vi "XMenuBar-Facade.vi"(0 "Data In":T5, 2 "Display State In":T3, 3 "Container State":T4) -> (6 "Data Out":T5, 7 "Display State Out":T3, 8 "Action":T2)   [LabVIEW 2020, in "XMenuBar.xctl"]
uses:
  XMenuBar.xctl
  XMenuBar-Data.ctl
  CMenu/CMenu.lvclass
  <vilib>/_xctls/Container State.ctl
  XMenuBar-State.ctl
  <vilib>/_xctls/Action.ctl
  Ctrls/black-Sel.ctl
  XSubMenu/XSubMenu.xctl
  <vilib>/_xctls/XControlSupport.lvlib
panel:
  in  "XSubMenu2":i32(xcontrol)
  in  "XSubMenu":i32(xcontrol)
  in  "Sel":T1
  out "MenuBar":string[](array[string])
  in  "BarBg":bool
  # "1. Drop the controls that make up the appearance\nof the XControl here.\n\n2. Resize the window to fit the controls\n\n3. If the XControl is of fixed size,  make the \n window not resizable from VI Properties->Window Appearance.\n\n4. If you want the controls to automatically size when the XControl sizes, check  \"Scale all objects on front panel when window resizes\" in File->VI Properties->Window Size page.\n\n5. Show the block diagram and handle events for the controls on this panel."
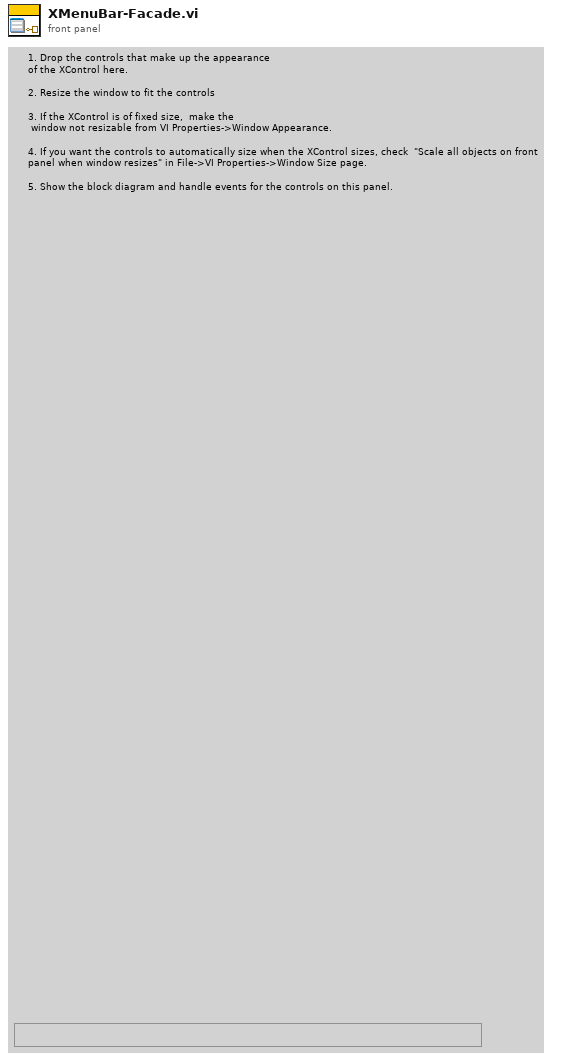
[diagram p1: front panel]
types:
  T1 = typedef "black-Sel.ctl" = bool
  T2 = typedef "XControlSupport.lvlib/Action.ctl" = cluster{"Data Changed?":bool, "State Changed?":bool, "Action Name":string}
  T3 = typedef "XMenuBar.xctl/XMenuBar-State.ctl" = cluster{"MenuFilePath":path}
  T4 = typedef "XControlSupport.lvlib/Container State.ctl" = cluster{"Indicator?":bool, "Run Mode?":bool, " Refnum":refnum<vi>}
  T5 = typedef "XMenuBar.xctl/XMenuBar-Data.ctl" = refnum<class "CMenu.lvclass">
  T6 = cluster{"Tag":string, "Name":string, "Symbol":i32, "Checked":bool, "ParentTag":string}[]
  T7 = enum16{"open", "replace", "create", "open or create", "replace or create", "replace or create with confirmation"}
  T8 = cluster{"Tag":string, "Name":string, "Symbol":i32, "Checked":bool, "ParentTag":string}
  T9 = cluster{"Tag":string, "Caption":string, "Symbol":i32, "Checked":bool, "OwnerTag":string}[]
  T10 = cluster{"Tag":string, "Name":string, "Index":i32, "Checked":bool, "Parent":string}[]
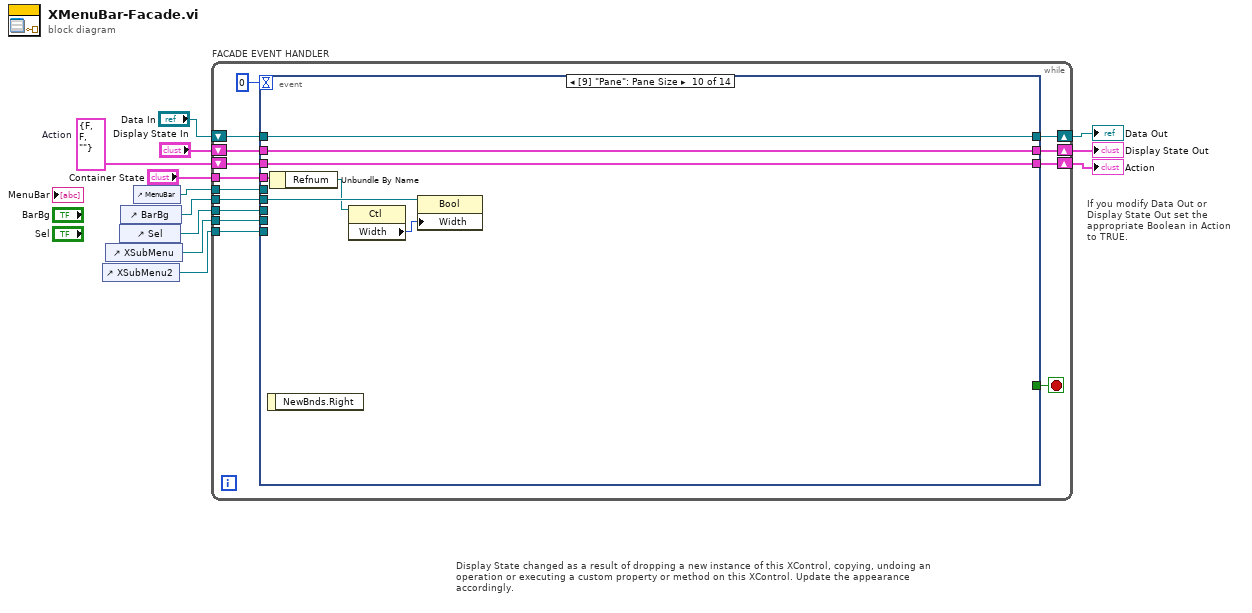
[diagram p0: block diagram]
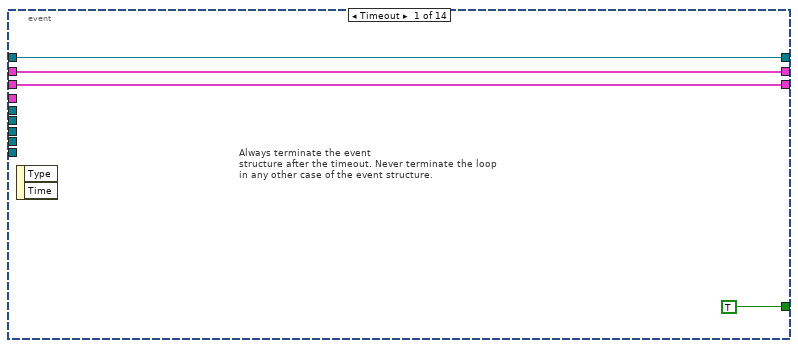
[diagram p2: hidden frame]
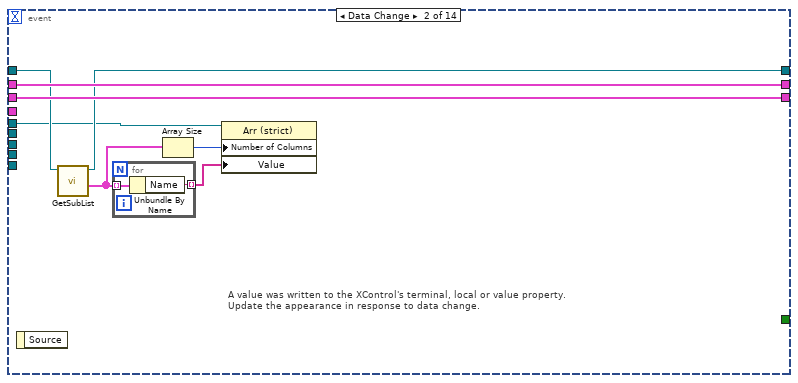
[diagram p3: hidden frame]
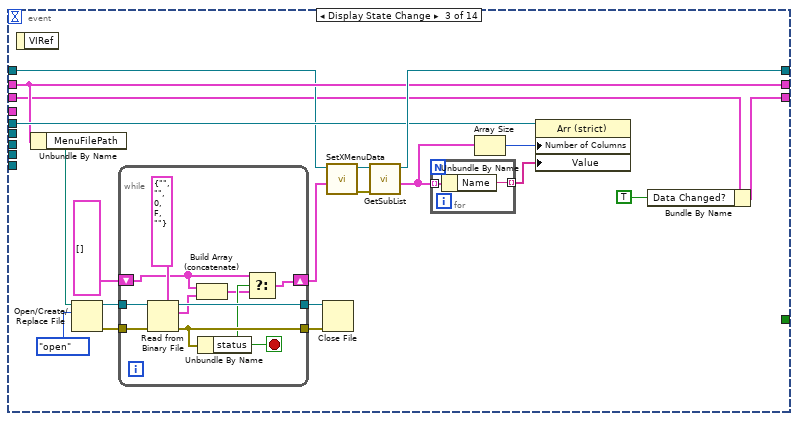
[diagram p4: hidden frame]
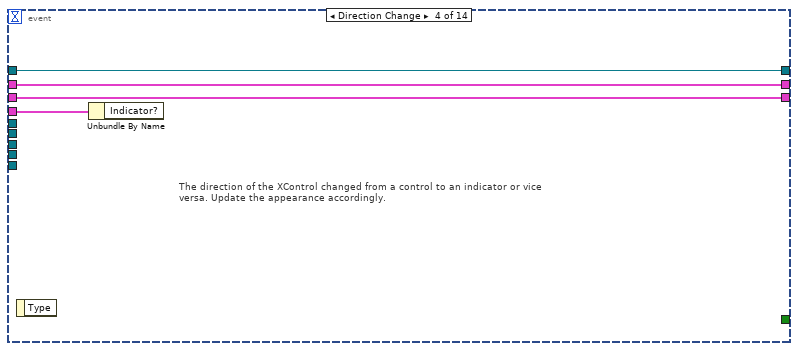
[diagram p5: hidden frame]
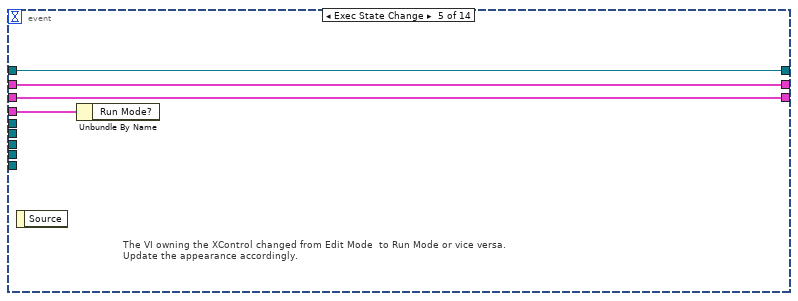
[diagram p6: hidden frame]
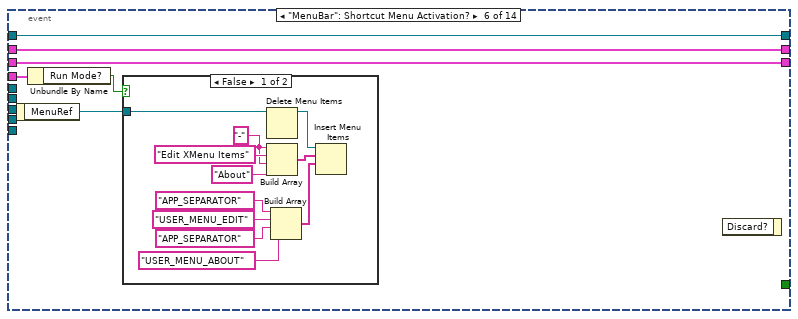
[diagram p7: hidden frame]
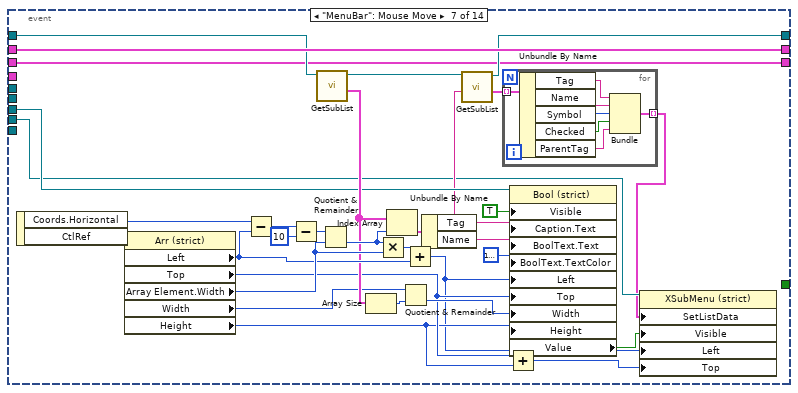
[diagram p9: hidden frame]
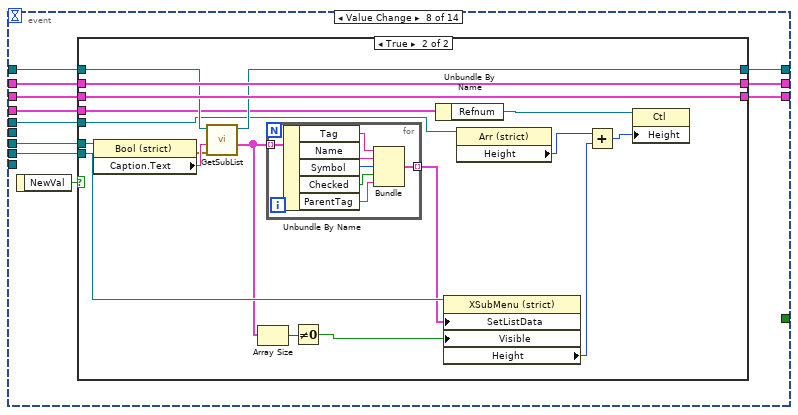
[diagram p10: hidden frame]
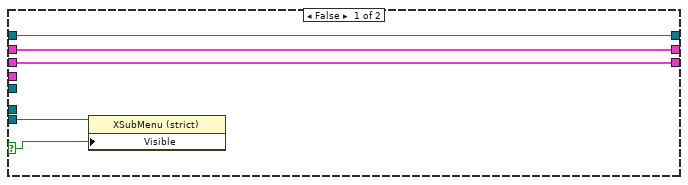
[diagram p11: hidden frame]
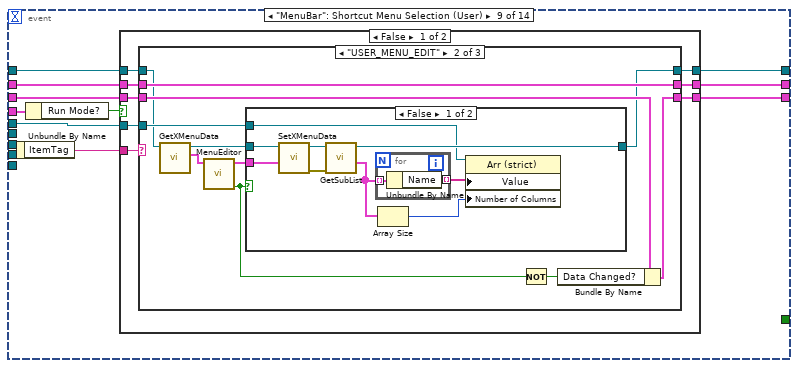
[diagram p12: hidden frame]
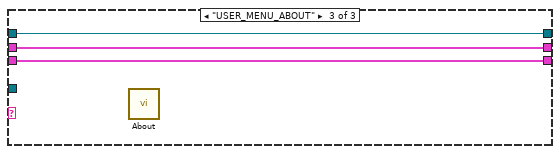
[diagram p15: hidden frame]
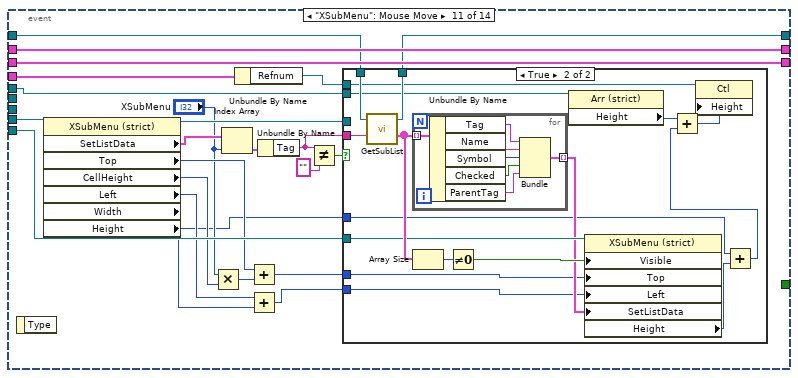
[diagram p17: hidden frame]
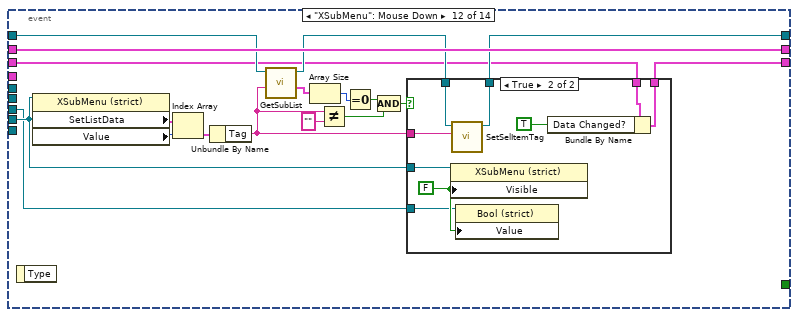
[diagram p19: hidden frame]
diagram:
  w6 = T2 {"Data Changed?"=FALSE, "State Changed?"=FALSE, "Action Name"=""}  # Action
  # "Display State changed as a result of dropping a new instance of this XControl, copying, undoing an operation or executing a custom property or method on this XControl. Update the appearance accordingly."
  # "If you modify Data Out or\nDisplay State Out set the\nappropriate Boolean in Action\nto TRUE."
  n1 = control-ref of="XSubMenu2"() -> (w1:refnum<vi>)
  n2 = control-ref of="XSubMenu"() -> (w2:refnum<vi>)
  n3 = control-ref of="Sel"() -> (w3:refnum<vi>)
  n4 = control-ref of="BarBg"() -> (w4:refnum<vi>)
  n5 = control-ref of="MenuBar"() -> (w5:refnum<vi>)
  n6 = while "FACADE EVENT HANDLER" {
    shift-right: [w25] -> w9
    shift-left: "Display State In" -> [w26]
    tunnel: "Container State" -> [w22]
    shift-right: [w20] -> w12
    shift-left: "Data In" -> [w21]
    shift-right: [w18] -> w7
    shift-left: w6 -> [w19]
    tunnel: w5 -> [w17]
    tunnel: w4 -> [w16]
    tunnel: w3 -> [w15]
    tunnel: w2 -> [w14]
    tunnel: w1 -> [w13]
    stop <- w24 stop-if-true
    n7 = event shown="[9] \"Pane\": Pane Size" {
      selector: _ -> [_ _ _ _ _ _ _ _ _ _ _ _ _ _]
      dyn-events: _ -> [_ _ _ _ _ _ _ _ _ _ _ _ _ _]
      timeout: 0 -> [_ _ _ _ _ _ _ _ _ _ _ _ _ _]
      tunnel: w26 -> [w28 w38 w52 w75 w79 w85 w129 w142 w182 w232 w258 w301 w326 w335]
      tunnel: [w28 w38 w52 w75 w79 w85 w129 w145 w181 w232 w258 w301 w326 w335] -> w25
      tunnel: [TRUE _ _ _ _ _ _ _ _ _ _ _ _ _] -> w24
      tunnel: w22 -> [_ _ _ w76 w80 w82 _ w138 w180 w230 w238 _ _ w330]
      tunnel: w21 -> [w27 w36 w46 w74 w78 w86 w122 w147 w186 w233 w252 w292 w320 w336]
      tunnel: [w27 w35 w59 w74 w78 w86 w106 w146 w185 w233 w251 w289 w319 w336] -> w20
      tunnel: [w29 w37 w42 w73 w77 w84 w99 w143 w183 w231 w257 w285 w317 w334] -> w18
      tunnel: w19 -> [w29 w37 w43 w73 w77 w84 w99 w144 w184 w231 w257 w286 w318 w334]
      tunnel: w17 -> [_ w34 w58 _ _ _ _ w137 w178 _ w236 _ _ w328]
      tunnel: w16 -> [_ _ _ _ _ _ _ _ _ w234 _ _ _ _]
      tunnel: w15 -> [_ _ _ _ _ _ w110 w141 _ _ _ w284 w314 _]
      tunnel: w14 -> [_ _ _ _ _ _ w101 w139 _ _ w249 w287 w315 w333]
      tunnel: w13 -> [_ _ _ _ _ _ _ _ _ _ w248 _ w325 w332]
      event Timeout {
        # "Always terminate the event\nstructure after the timeout. Never terminate the loop in any other case of the event structure."
        n8 = event-data() -> ()  [unwired: 1 in, 2 out]
      }
      event Data Change {
        # "A value was written to the XControl's terminal, local or value property.\nUpdate the appearance in response to data change."
        n9 = event-data() -> ()  [unwired: 1 in, 1 out]
        n10 = call "GetSubList.vi"("CMenu in"=w36) -> ("SubList"=w33:T6, "CMenu out"=w35:T5)  [unwired: 8 in, 1 out]
        n11 = for {
          tunnel: w33 -> [w40] mode=indexing
          tunnel: [w39] -> w31 mode=indexing
          n12 = Unbundle By Name(w40) -> ("Name"=w39:string)
        }
        n13 = Array Size(array=w33) -> (size(s)=w32:i32)
        n14 = property class="Arr (strict)"(reference=w34, "Number of Columns"=w32, "Value"=w31) -> ()  [unwired: 1 in, 2 out]
      }
      event Display State Change {
        n15 = event-data() -> ()  [unwired: 1 in, 1 out]
        n16 = Unbundle By Name(w52) -> ("MenuFilePath"=w51:path)
        n17 = Open/Create/Replace File(file path (use dialog)=w51, operation (0:open)=T7."open") -> (refnum out=w54:refnum<file>, error out=w53:errorcluster)  [unwired: 4 in, 1 out]
        n18 = while {
          tunnel: w54 -> [w69]
          tunnel: w53 -> [w68]
          tunnel: [w67] -> w50
          tunnel: [w66] -> w49
          shift-right: [w62] -> w47
          shift-left: T6 [] -> [w61]
          stop <- w65 stop-if-true
          n19 = Read from Binary File(5:T8 {"Tag"="", "Name"="", "Symbol"=0, "Checked"=FALSE, "ParentTag"=""} ("Item"), 8:w68, 11:w69) -> (0:w66:errorcluster, 2:w64:T8, 3:w67:refnum<file>)  [unwired: 3 in, 1 out]
          n20 = Build Array (concatenate)(w61, w64) -> (w63:T6)
          n21 = Unbundle By Name(w66) -> ("status"=w65:bool)
          n22 = Select(t=w61, s=w65, f=w63) -> (s? t:f=w62:T6)
        }
        n23 = Close File(refnum=w50, error in=w49) -> ()  [unwired: 2 out]
        n24 = call "SetXMenuData.vi"("Items"=w47, "CMenu in"=w46) -> ("error out"=w44:errorcluster, "CMenu out"=w45:T5)  [unwired: 8 in]
        n25 = call "GetSubList.vi"("error in (no error)"=w44, "CMenu in"=w45) -> ("SubList"=w57:T6, "CMenu out"=w59:T5)  [unwired: 7 in, 1 out]
        n26 = for {
          tunnel: w57 -> [w72] mode=indexing
          tunnel: [w71] -> w56 mode=indexing
          n27 = Unbundle By Name(w72) -> ("Name"=w71:string)
        }
        n28 = Array Size(array=w57) -> (size(s)=w60:i32)
        n29 = property class="Arr (strict)"(reference=w58, "Number of Columns"=w60, "Value"=w56) -> ()  [unwired: 1 in, 2 out]
        n30 = Bundle By Name(cluster=w43, "Data Changed?"=TRUE) -> (w42:T2)
      }
      event Direction Change {
        # "The direction of the XControl changed from a control to an indicator or vice versa. Update the appearance accordingly."
        n31 = event-data() -> ()  [unwired: 1 in, 1 out]
        n32 = Unbundle By Name(w76) -> ()  [unwired: 1 out]
      }
      event Exec State Change {
        # "The VI owning the XControl changed from Edit Mode  to Run Mode or vice versa.\nUpdate the appearance accordingly."
        n33 = event-data() -> ()  [unwired: 1 in, 1 out]
        n34 = Unbundle By Name(w80) -> ()  [unwired: 1 out]
      }
      event "MenuBar": Shortcut Menu Activation? {
        n35 = event-data() -> ("MenuRef"=w83:refnum<k9>)  [unwired: 1 in]
        n36 = Unbundle By Name(w82) -> ("Run Mode?"=w81:bool)
        n37 = case shown="False" w81 {
          tunnel: w83 -> [w91 _]
          frame False {
            w88 = "-"
            n38 = Delete Menu Items(9:w91) -> (3:w93:refnum<k9>)  [unwired: 3 in, 1 out]
            n39 = Build Array(w88, "Edit XMenu Items" ("element"), w88, "About" ("element")) -> (w97:string[])
            n40 = Build Array("APP_SEPARATOR", "USER_MENU_EDIT" ("element"), "APP_SEPARATOR" ("element"), "USER_MENU_ABOUT" ("element")) -> (w96:string[])
            n41 = Insert Menu Items(7:w96, 8:w97, 9:w93) -> ()  [unwired: 3 in, 3 out]
          }
          frame True {
          }
        }
        n42 = event-data() -> ()  [unwired: 2 in, 1 out]
      }
      event "MenuBar": Mouse Move {
        n43 = event-data() -> ("Coords.Horizontal"=w124:i32, "CtlRef"=w125:refnum<vi>)  [unwired: 1 in]
        n44 = property class="Arr (strict)"(reference=w125) -> ("Left"=w120:i32, "Top"=w109:i32, "Array Element.Width"=w121:u32, "Width"=w113:u32, "Height"=w108:u32)  [unwired: 1 in, 2 out]
        n45 = Subtract(x=w124, y=w120) -> (x-y=w126:i32)
        n46 = Subtract(x=w126, y=10) -> (x-y=w128:i32)
        n47 = call "GetSubList.vi"("CMenu in"=w122) -> ("SubList"=w117:T6, "CMenu out"=w107:T5)  [unwired: 8 in, 1 out]
        n48 = Quotient & Remainder(x=w128, y=w121) -> (floor(x/y)=w119:u32)  [unwired: 1 out]
        n49 = Array Size(array=w117) -> (size(s)=w116:i32)
        n50 = Multiply(x=w119, y=w121) -> (x*y=w127:u32)
        n51 = Index Array(array=w117, index=w119) -> (element=w118:T8)
        n52 = Quotient & Remainder(x=w113, y=w116) -> (floor(x/y)=w112:u32)  [unwired: 1 out]
        n53 = Add(x=w127, y=w120) -> (x+y=w103:u32)
        n54 = Unbundle By Name(w118) -> ("Tag"=w105:string, "Name"=w115:string)
        n55 = call "GetSubList.vi"("ParentTag(Empty for Top)"=w105, "CMenu in"=w107) -> ("SubList"=w104:T6, "CMenu out"=w106:T5)  [unwired: 7 in, 1 out]
        n56 = for {
          tunnel: w104 -> [w136] mode=indexing
          tunnel: [w133] -> w98 mode=indexing
          n57 = Unbundle By Name(w136) -> ("Tag"=w134:string, "Name"=w135:string, "Symbol"=w132:i32, "Checked"=w131:bool, "ParentTag"=w130:string)
          n58 = Bundle("Tag"=w134, "Name"=w135, "Symbol"=w132, "Checked"=w131, "ParentTag"=w130) -> (w133:T8)  [unwired: 1 in]
        }
        n59 = Add(x=w109, y=w108) -> (x+y=w102:u32)
        n60 = property class="Bool (strict)"(reference=w110, "Visible"=TRUE, "Caption.Text"=w105, "BoolText.Text"=w115, "BoolText.TextColor"=u32 16777226, "Left"=w103, "Top"=w109, "Width"=w112, "Height"=w108) -> ("Value"=w100:bool)  [unwired: 1 in, 2 out]
        n61 = property class="XSubMenu (strict)"(reference=w101, "SetListData"=w98, "Visible"=w100, "Left"=w103, "Top"=w102) -> ()  [unwired: 1 in, 2 out]
      }
      event Value Change {
        n62 = event-data() -> ("NewVal"=w140:T1)  [unwired: 1 in]
        n63 = case shown="True" w140 {
          selector: w140 -> [w148 _]
          tunnel: [w152 w165] -> w146
          tunnel: w147 -> [w152 w166]
          tunnel: [w151 w170] -> w145
          tunnel: [w150 w169] -> w143
          tunnel: w144 -> [w150 w169]
          tunnel: w142 -> [w151 w170]
          tunnel: w141 -> [_ w168]
          tunnel: w139 -> [w149 w163]
          tunnel: w138 -> [_ w158]
          tunnel: w137 -> [_ w154]
          frame False {
            n64 = property class="XSubMenu (strict)"(reference=w149, "Visible"=w148) -> ()  [unwired: 1 in, 2 out]
          }
          frame True {
            n65 = property class="Bool (strict)"(reference=w168) -> (error out=w164:errorcluster, "Caption.Text"=w167:string)  [unwired: 1 in, 1 out]
            n66 = call "GetSubList.vi"("error in (no error)"=w164, "ParentTag(Empty for Top)"=w167, "CMenu in"=w166) -> ("SubList"=w160:T6, "CMenu out"=w165:T5)  [unwired: 6 in, 1 out]
            n67 = Array Size(array=w160) -> (size(s)=w162:i32)
            n68 = for {
              tunnel: w160 -> [w177] mode=indexing
              tunnel: [w174] -> w159 mode=indexing
              n69 = Unbundle By Name(w177) -> ("Tag"=w175:string, "Name"=w176:string, "Symbol"=w173:i32, "Checked"=w172:bool, "ParentTag"=w171:string)
              n70 = Bundle("Tag"=w175, "Name"=w176, "Symbol"=w173, "Checked"=w172, "ParentTag"=w171) -> (w174:T8)  [unwired: 1 in]
            }
            n71 = Not Equal To 0?(x=w162) -> (x != 0?=w161:bool)
            n72 = Unbundle By Name(w158) -> ("Refnum"=w155:refnum<vi>)
            n73 = property class="XSubMenu (strict)"(reference=w163, "SetListData"=w159, "Visible"=w161) -> ("Height"=w157:u32)  [unwired: 1 in, 2 out]
            n74 = property class="Arr (strict)"(reference=w154) -> ("Height"=w153:u32)  [unwired: 1 in, 2 out]
            n75 = Add(x=w153, y=w157) -> (x+y=w156:u32)
            n76 = property class="Ctl"(reference=w155, "Height"=w156) -> ()  [unwired: 1 in, 2 out]
          }
        }
      }
      event "MenuBar": Shortcut Menu Selection (User) {
        n77 = event-data() -> ("ItemTag"=w187:string)  [unwired: 1 in]
        n78 = Unbundle By Name(w180) -> ("Run Mode?"=w179:bool)
        n79 = case shown="False" w179 {
          tunnel: w187 -> [w195 _]
          tunnel: w186 -> [w194 w227]
          tunnel: [w193 w227] -> w185
          tunnel: w184 -> [w192 w225]
          tunnel: [w191 w225] -> w183
          tunnel: w182 -> [w190 w226]
          tunnel: [w189 w226] -> w181
          tunnel: w178 -> [w188 _]
          frame False {
            n80 = case shown="\"USER_MENU_EDIT\"" w195 {
              tunnel: w194 -> [w198 w200 w224]
              tunnel: [w198 w204 w224] -> w193
              tunnel: w192 -> [w196 w208 w222]
              tunnel: [w196 w207 w222] -> w191
              tunnel: w190 -> [w197 w206 w223]
              tunnel: [w197 w206 w223] -> w189
              tunnel: w188 -> [_ w202 _]
              frame Default {
              }
              frame "USER_MENU_EDIT" {
                n81 = call "GetXMenuData.vi"("CMenu in"=w200) -> ("Items"=w201:T9, "CMenu out"=w199:T5)  [unwired: 8 in, 1 out]
                n82 = call "MenuEditor.vi"("ItemsIn"=w201) -> ("Cancelled?"=w203:bool, "ItemsOut"=w205:T10)  [unwired: 9 in]
                n83 = case shown="False" w203 {
                  tunnel: w199 -> [w218 w221]
                  tunnel: w205 -> [w217 _]
                  tunnel: [w214 w221] -> w204
                  tunnel: w202 -> [w213 _]
                  frame False {
                    n84 = call "SetXMenuData.vi"("Items"=w217, "CMenu in"=w218) -> ("error out"=w215:errorcluster, "CMenu out"=w216:T5)  [unwired: 8 in]
                    n85 = call "GetSubList.vi"("error in (no error)"=w215, "CMenu in"=w216) -> ("SubList"=w211:T6, "CMenu out"=w214:T5)  [unwired: 7 in, 1 out]
                    n86 = for {
                      tunnel: w211 -> [w220] mode=indexing
                      tunnel: [w219] -> w212 mode=indexing
                      n87 = Unbundle By Name(w220) -> ("Name"=w219:string)
                    }
                    n88 = Array Size(array=w211) -> (size(s)=w210:i32)
                    n89 = property class="Arr (strict)"(reference=w213, "Value"=w212, "Number of Columns"=w210) -> ()  [unwired: 1 in, 2 out]
                  }
                  frame True {
                  }
                }
                n90 = Not(x=w203) -> (.not. x?=w209:bool)
                n91 = Bundle By Name(cluster=w208, "Data Changed?"=w209) -> (w207:T2)
              }
              frame "USER_MENU_ABOUT" {
                n92 = call "About.vi"() -> ()  [unwired: 12 in]
              }
            }
          }
          frame True {
            # "Disable Runtime Menu"
          }
        }
      }
      event Pane Size {
        n93 = event-data() -> ()  [unwired: 1 in, 1 out]
        n94 = Unbundle By Name(w230) -> ("Refnum"=w229:refnum<vi>)
        n95 = property class="Ctl"(reference=w229) -> ("Width"=w228:u32)  [unwired: 1 in, 2 out]
        n96 = property class="Bool"(reference=w234, "Width"=w228) -> ()  [unwired: 1 in, 2 out]
      }
      event "XSubMenu": Mouse Move {
        n97 = event-data() -> ()  [unwired: 1 in, 1 out]
        n98 = property class="XSubMenu (strict)"(reference=w249) -> (reference out=w250:refnum<vi>, "SetListData"=w255:T6, "Top"=w247:i32, "CellHeight"=w244:i32, "Left"=w242:i32, "Width"=w241:u32, "Height"=w235:u32)  [unwired: 1 in, 1 out]
        n99 = Multiply(x="XSubMenu", y=w244) -> (x*y=w246:i32)
        n100 = Index Array(array=w255, index="XSubMenu") -> (element=w256:T8)
        n101 = Unbundle By Name(w238) -> ("Refnum"=w237:refnum<vi>)
        n102 = Add(x=w247, y=w246) -> (x+y=w243:i32)
        n103 = Add(x=w242, y=w241) -> (x+y=w240:u32)
        n104 = Unbundle By Name(w256) -> ("Tag"=w239:string)
        n105 = Not Equal?(x=w239, y="") -> (x != y?=w253:bool)
        n106 = case shown="True" w253 {
          tunnel: w252 -> [w259 w276]
          tunnel: [w259 w275] -> w251
          tunnel: w250 -> [_ _]
          tunnel: w248 -> [_ w272]
          tunnel: w243 -> [_ w263]
          tunnel: w240 -> [_ w269]
          tunnel: w239 -> [_ w268]
          tunnel: w237 -> [_ w266]
          tunnel: w236 -> [_ w265]
          tunnel: w235 -> [_ w262]
          frame False {
          }
          frame True {
            n107 = call "GetSubList.vi"("ParentTag(Empty for Top)"=w268, "CMenu in"=w276) -> ("SubList"=w273:T6, "CMenu out"=w275:T5)  [unwired: 7 in, 1 out]
            n108 = for {
              tunnel: w273 -> [w283] mode=indexing
              tunnel: [w280] -> w270 mode=indexing
              n109 = Unbundle By Name(w283) -> ("Tag"=w281:string, "Name"=w282:string, "Symbol"=w279:i32, "Checked"=w278:bool, "ParentTag"=w277:string)
              n110 = Bundle("Tag"=w281, "Name"=w282, "Symbol"=w279, "Checked"=w278, "ParentTag"=w277) -> (w280:T8)  [unwired: 1 in]
            }
            n111 = Array Size(array=w273) -> (size(s)=w274:i32)
            n112 = Not Equal To 0?(x=w274) -> (x != 0?=w271:bool)
            n113 = property class="Arr (strict)"(reference=w265) -> ("Height"=w264:u32)  [unwired: 1 in, 2 out]
            n114 = property class="XSubMenu (strict)"(reference=w272, "Visible"=w271, "Top"=w263, "Left"=w269, "SetListData"=w270) -> ("Height"=w261:u32)  [unwired: 1 in, 2 out]
            n115 = Add(x=w262, y=w261) -> (x+y=w260:u32)
            n116 = Add(x=w264, y=w260) -> (x+y=w267:u32)
            n117 = property class="Ctl"(reference=w266, "Height"=w267) -> ()  [unwired: 1 in, 2 out]
          }
        }
      }
      event "XSubMenu": Mouse Down {
        n118 = event-data() -> ()  [unwired: 1 in, 1 out]
        n119 = property class="XSubMenu (strict)"(reference=w287) -> ("SetListData"=w299:T6, "Value"=w298:i32)  [unwired: 1 in, 2 out]
        n120 = Index Array(array=w299, index=w298) -> (element=w300:T8)
        n121 = Unbundle By Name(w300) -> ("Tag"=w288:string)
        n122 = call "GetSubList.vi"("ParentTag(Empty for Top)"=w288, "CMenu in"=w292) -> ("SubList"=w296:T6, "CMenu out"=w290:T5)  [unwired: 7 in, 1 out]
        n123 = Array Size(array=w296) -> (size(s)=w295:i32)
        n124 = Not Equal?(x=w288, y="") -> (x != y?=w294:bool)
        n125 = Equal To 0?(x=w295) -> (x = 0?=w293:bool)
        n126 = Compound Arithmetic op=AND(w293, w294) -> (w291:bool)
        n127 = case shown="True" w291 {
          tunnel: w290 -> [w303 w312]
          tunnel: [w303 w311] -> w289
          tunnel: w288 -> [_ w310]
          tunnel: w287 -> [_ w309]
          tunnel: w286 -> [w302 w307]
          tunnel: [w302 w306] -> w285
          tunnel: w284 -> [_ w304]
          frame False {
          }
          frame True {
            w305 = FALSE ("Visible")
            n128 = property class="XSubMenu (strict)"(reference=w309, "Visible"=w305) -> ()  [unwired: 1 in, 2 out]
            n129 = call "SetSelItemTag.vi"("SelItemTag"=w310, "CMenu in"=w312) -> ("CMenu out"=w311:T5)  [unwired: 8 in, 1 out]
            n130 = property class="Bool (strict)"(reference=w304, "Value"=w305) -> ()  [unwired: 1 in, 2 out]
            n131 = Bundle By Name(cluster=w307, "Data Changed?"=TRUE) -> (w306:T2)
          }
        }
      }
      event "XSubMenu2": Mouse Down {
        w313 = FALSE ("Visible")
        n132 = event-data() -> ()  [unwired: 1 in, 1 out]
        n133 = property class="XSubMenu (strict)"(reference=w325, "Visible"=w313) -> ("SetListData"=w324:T6)  [unwired: 1 in, 2 out]
        n134 = property class="XSubMenu (strict)"(reference=w315, "Visible"=w313) -> ()  [unwired: 1 in, 2 out]
        n135 = property class="Bool (strict)"(reference=w314, "Value"=w313) -> ()  [unwired: 1 in, 2 out]
        n136 = Index Array(array=w324, index="XSubMenu2") -> (element=w322:T8)
        n137 = Unbundle By Name(w322) -> ("Tag"=w321:string)
        n138 = call "SetSelItemTag.vi"("SelItemTag"=w321, "CMenu in"=w320) -> ("CMenu out"=w319:T5)  [unwired: 8 in, 1 out]
        n139 = Bundle By Name(cluster=w318, "Data Changed?"=TRUE) -> (w317:T2)
      }
      event Mouse Down {
        w331 = FALSE ("Visible")
        n140 = event-data() -> ()  [unwired: 1 in, 1 out]
        n141 = property class="XSubMenu (strict)"(reference=w333, "Visible"=w331) -> ()  [unwired: 1 in, 2 out]
        n142 = property class="XSubMenu (strict)"(reference=w332, "Visible"=w331) -> ()  [unwired: 1 in, 2 out]
        n143 = Unbundle By Name(w330) -> ("Refnum"=w329:refnum<vi>)
        n144 = property class="Arr (strict)"(reference=w328) -> ("Height"=w327:u32)  [unwired: 1 in, 2 out]
        n145 = property class="Ctl"(reference=w329, "Height"=w327) -> ()  [unwired: 1 in, 2 out]
      }
    }
  }
  "Display State Out" <- w9
  "Data Out" <- w12
  "Action" <- w7
